vi "Test sort.vi"(11 "Error in":errorcluster) -> (15 "Error out":errorcluster)   [LabVIEW 2020, in "BubbleSort Tests.lvlib"]
doc: "This VI validates Bubble sort"
uses:
  BubbleSort Tests.lvlib
  <vilib>/SLL Drona/APIs/Stimulus/ControlValue/SetValueAuto.vi
  <vilib>/SLL Drona/APIs/Assert/AssertControlValue/Equal.vi
  <vilib>/SLL Drona/APIs/Stimulus/VI/CloseVI.vi
  <vilib>/Utility/error.llb/Error Cluster From Error Code.vi
  <vilib>/ErrorRing/Error Ring.xnode
  <vilib>/addons/_JKI Toolkits/Caraya/classes/Test/Test.lvclass
  <vilib>/SLL Drona/Drona.lvlib
  <vilib>/SLL Drona/APIs/Stimulus/ControlValue/ControlValue.lvlib
  <vilib>/SLL Drona/APIs/Assert/AssertControlValue/AssertControlValue.lvlib
  <vilib>/SLL Drona/APIs/Stimulus/VI/VI.lvlib
  <vilib>/Wiresmith Technology/G CLI/CLI Class/CLI.lvclass
panel:
  # "BUBBLE SORT TEST"
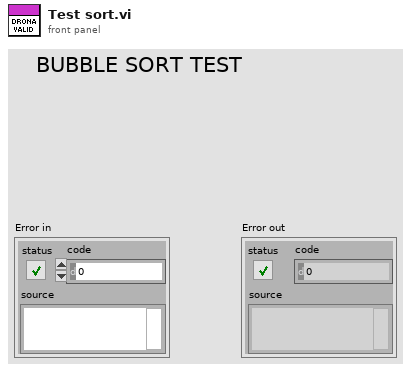
[diagram p1: front panel]
types:
  T1 = cluster{"Input Array":dbl[], "Sorting order":enum16{"Descending Order", "Ascending Order"}, "Output Array":dbl[]}[]
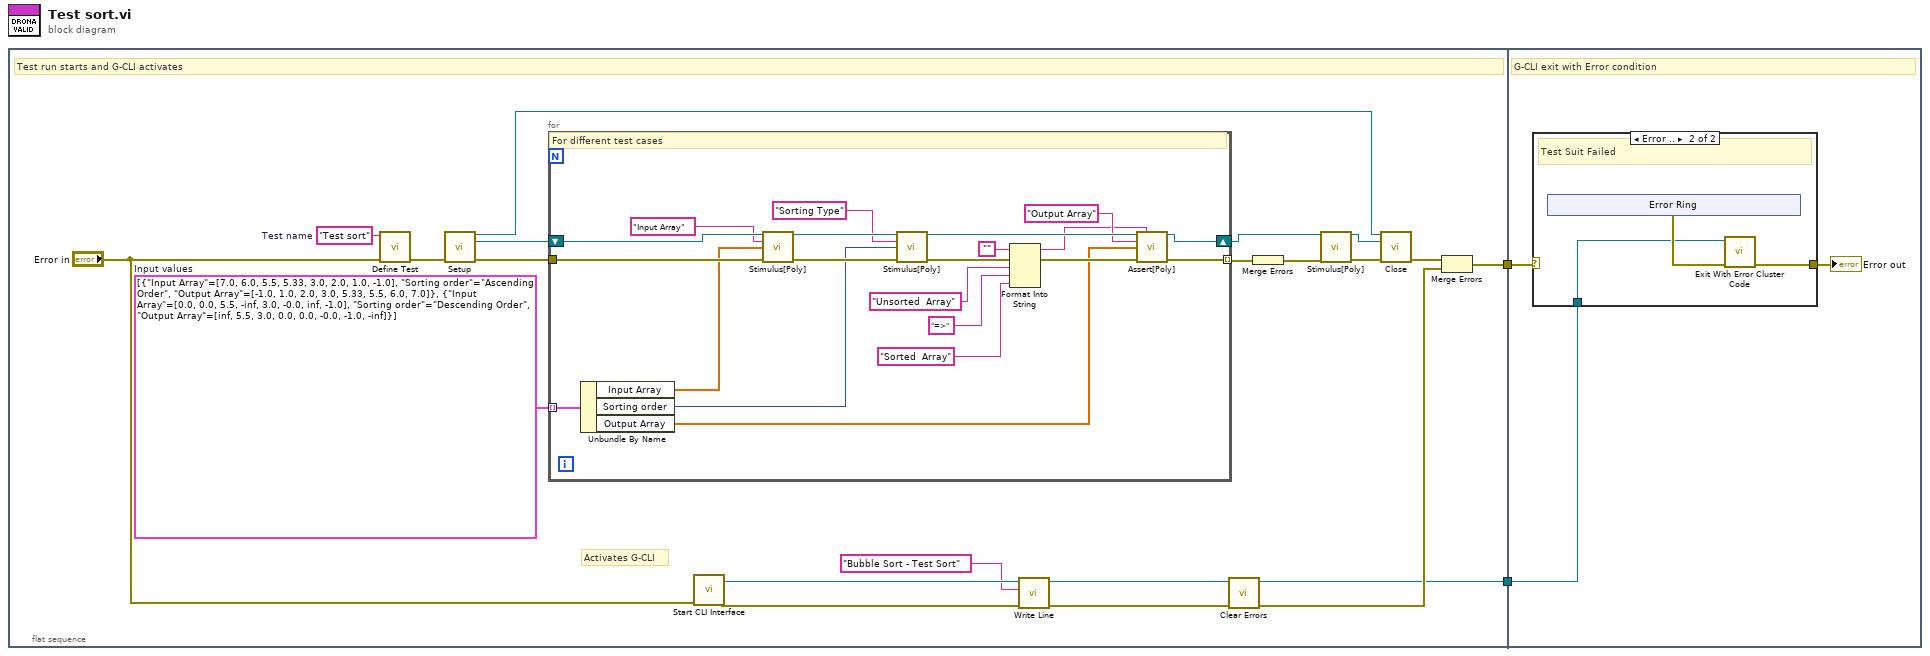
[diagram p0: block diagram]
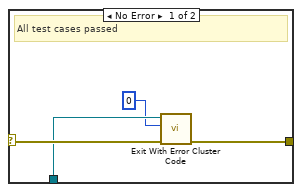
[diagram p2: hidden frame]
diagram:
  n1 = flat-sequence {
    tunnel: [w6] -> w2
    tunnel: [w3] -> w1
    tunnel: w2 -> [w46]
    tunnel: w1 -> [w45]
    frame #0 {
      w21 = T1 [{"Input Array"=[7.0, 6.0, 5.5, 5.33, 3.0, 2.0, 1.0, -1.0], "Sorting order"=enum."Ascending Order", "Output Array"=[-1.0, 1.0, 2.0, 3.0, 5.33, 5.5, 6.0, 7.0]}, {"Input Array"=[0.0, 0.0, 5.5, -inf, 3.0, -0.0, inf, -1.0], "Sorting order"=enum."Descending Order", "Output Array"=[inf, 5.5, 3.0, 0.0, 0.0, -0.0, -1.0, -inf]}]  # Input values
      w22 = "Test sort"  # Test name
      # "Activates G-CLI"
      # "Test run starts and G-CLI activates"
      n2 = call <vilib>:"Define Test.vi"("error in (no error)"="Error in", "Label (VI Title)"=w22) -> ("error out"=w20:errorcluster)  [unwired: 9 in]
      n3 = call <vilib>:"Setup.vi"("error in"=w20) -> ("Application Ref"=w17:refnum<vi>, "VI Reference Out"=w18:refnum<vi>, "error out"=w19:errorcluster)  [unwired: 12 in]
      n4 = for {
        tunnel: w21 -> [w42] mode=indexing
        shift-right: [w23] -> w15
        shift-left: w18 -> [w41]
        tunnel: w19 -> [w43]
        tunnel: [w32] -> w13 mode=indexing
        # "For different test cases"
        n5 = Unbundle By Name(w42) -> ("Input Array"=w27:dbl[], "Sorting order"=w38:enum16{"Descending Order", "Ascending Order"}, "Output Array"=w31:dbl[])
        n6 = call-poly <vilib>:"Stimulus[Poly].vi"("VI Reference In"=w41, "Control Path"="Input Array", "Value (Signaling)"=w27, "error in"=w43) -> ("VI Reference Out"=w37:refnum<vi>, "error out"=w39:errorcluster)  [unwired: 10 in]
        n7 = call-poly <vilib>:"Stimulus[Poly].vi"("VI Reference In"=w37, "Control Path"="Sorting Type", "Value (Signaling)"=w38, "error in"=w39) -> ("VI Reference Out"=w30:refnum<vi>, "error out"=w35:errorcluster)  [unwired: 10 in]
        n8 = Format Into String(initial string="", error in=w35, "Unsorted  Array" ("Control Path"), "=>" ("Control Path"), "Sorted  Array" ("Control Path")) -> (resulting string=w24:string, error out=w33:errorcluster)  [unwired: 1 in]
        n9 = call-poly <vilib>:"Assert[Poly].vi"("VI Reference In"=w30, "Test Label"=w24, "Control Path"="Output Array", "Control Value"=w31, "Error In"=w33) -> ("VI Reference Out"=w23:refnum<vi>, "Error Out"=w32:errorcluster)  [unwired: 9 in]
      }
      n10 = call <vilib>:"Start CLI Interface.vi"("error in (no error)"="Error in") -> ("error out"=w9:errorcluster, "CLI out"=w8:refnum<class "CLI.lvclass">)  [unwired: 7 in, 2 out]
      n11 = call <vilib>:"Write Line.vi"("error in (no error)"=w9, "Text to Write"="Bubble Sort - Test Sort", "CLI in"=w8) -> ("error out"=w5:errorcluster, "CLI out"=w3:refnum<class "CLI.lvclass">)  [unwired: 7 in]
      n12 = call <vilib>:"Clear Errors.vi"("error in (no error)"=w5) -> ("error out"=w4:errorcluster)  [unwired: 5 in, 1 out]
      n13 = Merge Errors(w13) -> (w12:errorcluster)
      n14 = call-poly <vilib>:"Stimulus[Poly].vi"("VI Reference In"=w15, "error in"=w12) -> ("VI Reference Out"=w14:refnum<vi>, "error out"=w16:errorcluster)  [unwired: 12 in]
      n15 = call <vilib>:"Close.vi"("Application Ref"=w17, "VI Reference"=w14, "error in"=w16) -> ("error out"=w11:errorcluster)  [unwired: 12 in]
      n16 = Merge Errors(w11, w4) -> (w6:errorcluster)
    }
    frame #1 {
      # "G-CLI exit with Error condition"
      n17 = case shown="Error .." w46 {
        selector: w46 -> [w50 _]
        tunnel: w45 -> [w49 w51]
        tunnel: [w47 w53] -> w44
        frame No Error {
          # "All test cases passed"
          n18 = call <vilib>:"Exit With Error Cluster Code.vi"("error in (no error)"=w50, "No Error Code (0)"=0, "CLI in"=w49) -> ("error out"=w47:errorcluster)  [unwired: 8 in]
        }
        frame Error {
          # "Test Suit Failed"
          n19 = xnode "Error Ring"() -> ("error out"=w52:errorcluster)
          n20 = call <vilib>:"Exit With Error Cluster Code.vi"("error in (no error)"=w52, "CLI in"=w51) -> ("error out"=w53:errorcluster)  [unwired: 9 in]
        }
      }
      "Error out" <- w44
    }
  }
